vi "genHelpFileIn.vi"(0 "Output Cluster":T1) -> (5 "Help Description":string="\n")   [LabVIEW 2017]
uses:
  <vilib>/express/express shared/propPageData.ctl
panel:
  in  "Start Row Data":string="Start Row Data:"
  in  "Samples":string="Samples:"
  in  "File Path":string="File Path:"
  in  "Attempt to Read Generic Text Files enum":string[](array[string])=["False", "True"]
  in  "Attempt to Read Generic Text Files":string="Read Generic Text Files:"
  in  "Lock File enum":string[](array[string])=[" False", " True"]
  in  "Lock File":string="Lock File:"
  in  "First Column enum":string[](array[string])=[" False", " True"]
  in  "First Column is Time Channel":string="First Column is Time  Channel: "
  in  "First Row enum":string[](array[string])=[" False", " True"]
  in  "First Row is Channel Names:":string="First Row is Channel: Names:"
  in  "Segment Size enum":string[](array[string])=["Retrieve segments of original size", "Retrieve segments of specified size"]
  in  "Segment Size":string="Segment Size: "
  in  "File_dialog enum":string[](array[string])=[" False", " True"]
  in  "File_dialog":string="Ask User To Choose File:"
  in  "Decimal enum":string[](array[string])=[". (dot)", ". (comma)"]
  in  "Decimal":string="Decimal Point: "
  in  "Timestamp":string="Timestamp: "
  in  "Timestamp enum":string[](array[string])=["Absolute", "Relative"]
  in  "Delimiter enum":string[](array[string])=["Tabulator", "Comma"]
  in  "Delimiter":string="Delimiter: "
  in  "Format enum":string[](array[string])=["Text (LVM)", "Binary with XML Header (TDM)", "Binary (TDMS)"]
  in  "Format":string="File Format: "
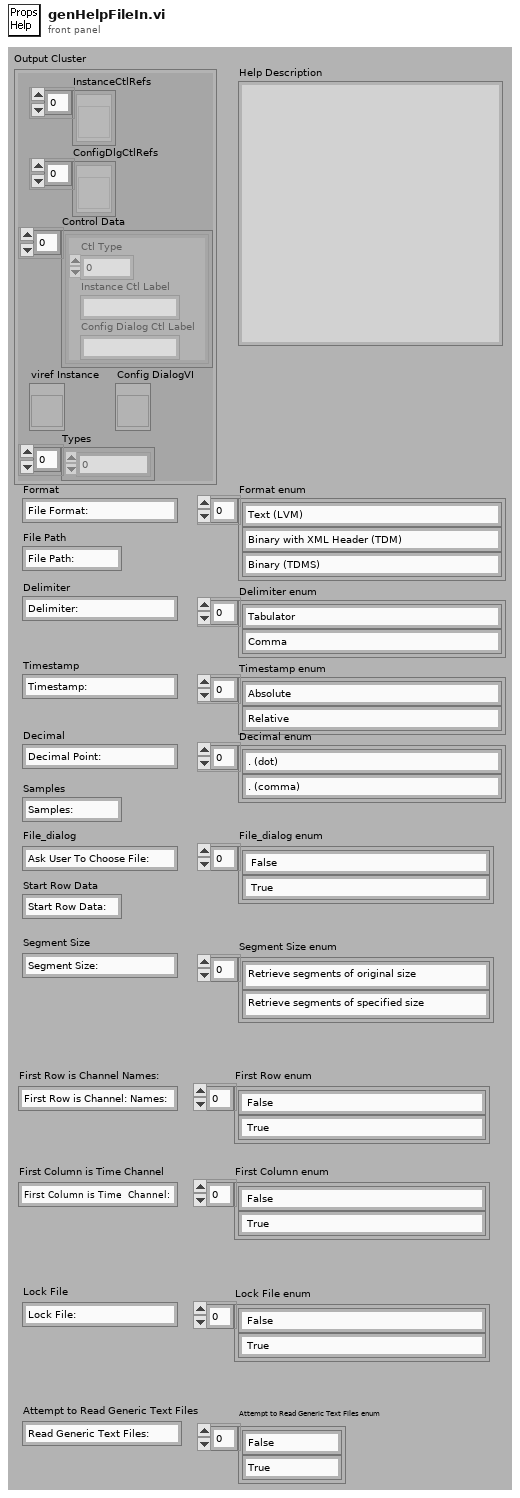
[diagram p1: front panel]
types:
  T1 = typedef "propPageData.ctl" = cluster{"InstanceCtlRefs":refnum<vi>[], "ConfigDlgCtlRefs":refnum<vi>[], "Control Data":cluster{"Ctl Type":u16, "Instance Ctl Label":string, "Config Dialog Ctl Label":string}[], "viref Instance":refnum<vi>, "Types":i32[], "Config DialogVI":refnum<vi>}
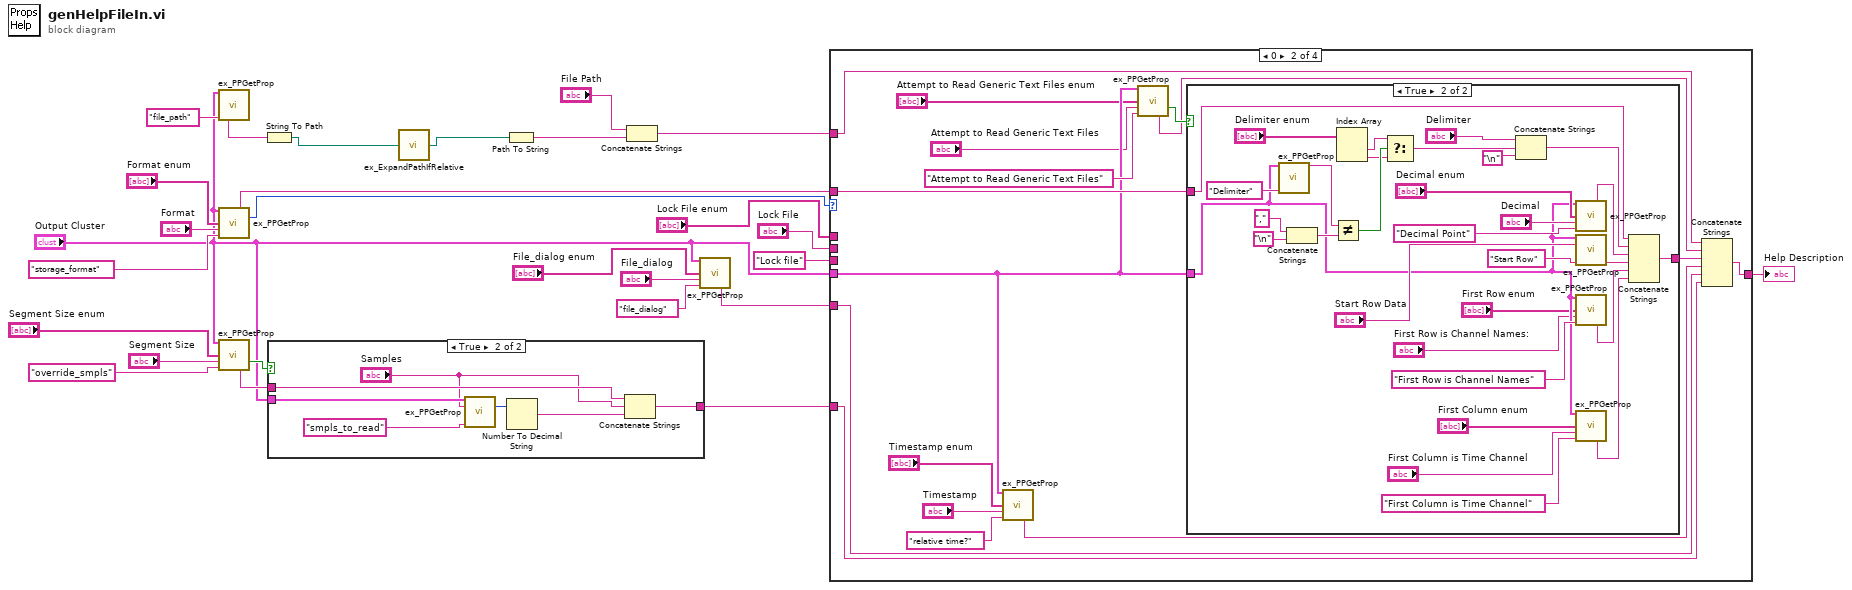
[diagram p0: block diagram]
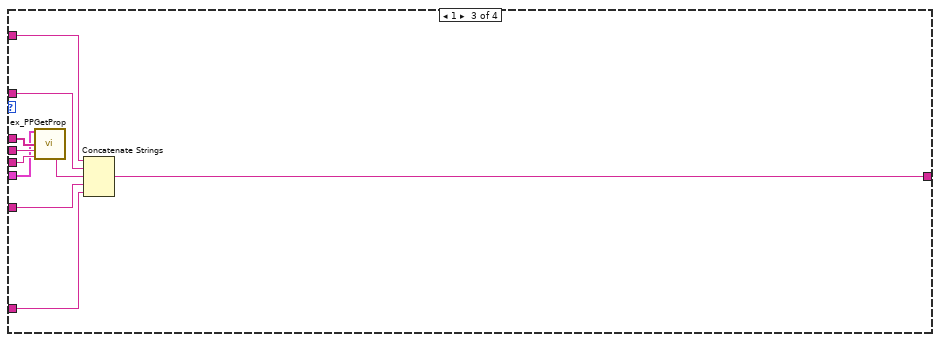
[diagram p5: hidden frame]
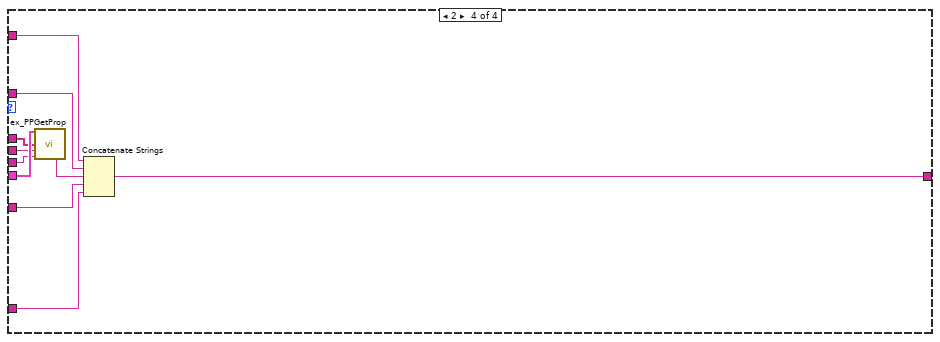
[diagram p6: hidden frame]
diagram:
  n1 = call <vilib>:"ex_PPGetProp.vi"("Output Cluster"="Output Cluster", "Control:"="file_path") -> ("String (Path)"=w6:string)  [unwired: 5 in, 8 out]
  n2 = call <vilib>:"ex_PPGetProp.vi"("Output Cluster"="Output Cluster", "Enum & T/F Strings"="Format enum", "Prefix"="Format", "Control:"="storage_format") -> ("Enum Result"=w24:string, "int32"=w23:i32)  [unwired: 3 in, 7 out]
  n3 = call <vilib>:"ex_PPGetProp.vi"("Output Cluster"="Output Cluster", "Enum & T/F Strings"="Segment Size enum", "Prefix"="Segment Size", "Control:"="override_smpls") -> ("bool"=w14:bool, "T/F Result"=w13:string)  [unwired: 3 in, 7 out]
  n4 = String To Path(string=w6) -> (path=w2:path)
  n5 = case shown="True" w14 {
    tunnel: [w28 w30] -> w12
    tunnel: w13 -> [w28 w32]
    tunnel: "Output Cluster" -> [_ w34]
    frame False {
    }
    frame True {
      n6 = call <vilib>:"ex_PPGetProp.vi"("Output Cluster"=w34, "Previous String"="Samples", "Control:"="smpls_to_read") -> ("int32"=w33:i32)  [unwired: 4 in, 8 out]
      n7 = Number To Decimal String(number=w33) -> (decimal integer string=w31:string)  [unwired: 1 in]
      n8 = Concatenate Strings(w32, "Samples", w31) -> (w30:string)
    }
  }
  n9 = call <vilib>:"ex_ExpandPathIfRelative.vi"("Path"=w2) -> ("Expanded path"=w1:path)  [unwired: 3 in, 1 out]
  n10 = Path To String(path=w1) -> (string=w5:string)
  n11 = Concatenate Strings("File Path", w5) -> (w3:string)
  n12 = call <vilib>:"ex_PPGetProp.vi"("Output Cluster"="Output Cluster", "Enum & T/F Strings"="File_dialog enum", "Prefix"="File_dialog", "Control:"="file_dialog") -> ("T/F Result"=w18:string)  [unwired: 3 in, 8 out]
  n13 = case shown="0" w23 {
    tunnel: "Output Cluster" -> [_ w44 w91 w104]
    tunnel: w24 -> [w36 w47 w90 w103]
    tunnel: [w36 w45 w86 w99] -> w22
    tunnel: w18 -> [_ w42 w88 w101]
    tunnel: w12 -> [_ w41 w87 w100]
    tunnel: "Lock File enum" -> [_ _ w94 w98]
    tunnel: "Lock File" -> [_ _ w93 w97]
    tunnel: "Lock file" -> [_ _ w92 w96]
    tunnel: w3 -> [_ w38 w85 w95]
    frame Default {
    }
    frame 0 {
      n14 = call <vilib>:"ex_PPGetProp.vi"("Output Cluster"=w44, "Enum & T/F Strings"="Timestamp enum", "Prefix"="Timestamp", "Control:"="relative time?") -> ("T/F Result"=w43:string)  [unwired: 3 in, 8 out]
      n15 = call <vilib>:"ex_PPGetProp.vi"("Output Cluster"=w44, "Enum & T/F Strings"="Attempt to Read Generic Text Files enum", "Prefix"="Attempt to Read Generic Text Files", "Control:"="Attempt to Read Generic Text Files") -> ("bool"=w51:bool, "T/F Result"=w37:string)  [unwired: 3 in, 7 out]
      n16 = case shown="True" w51 {
        tunnel: w44 -> [_ w60]
        tunnel: w47 -> [w53 w81]
        tunnel: [w53 w80] -> w46
        frame False {
        }
        frame True {
          n17 = call <vilib>:"ex_PPGetProp.vi"("Output Cluster"=w60, "Control:"="Delimiter") -> ("String"=w70:string)  [unwired: 5 in, 8 out]
          n18 = Concatenate Strings("," ("y"), "\n") -> (w69:string)
          n19 = Not Equal?(x=w70, y=w69) -> (x != y?=w77:bool)
          n20 = Index Array(array="Delimiter enum") -> (element #1=w75:string, element #2=w74:string)  [unwired: 2 in]
          n21 = Select(t=w75, s=w77, f=w74) -> (s? t:f=w73:string)
          n22 = Concatenate Strings("Delimiter", w73, "\n") -> (w71:string)
          n23 = call <vilib>:"ex_PPGetProp.vi"("Output Cluster"=w60, "Enum & T/F Strings"="Decimal enum", "Prefix"="Decimal", "Control:"="Decimal Point") -> ("Enum Result"=w79:string)  [unwired: 3 in, 8 out]
          n24 = call <vilib>:"ex_PPGetProp.vi"("Output Cluster"=w60, "Previous String"="Start Row Data", "Control:"="Start Row") -> ("dbl String"=w64:string)  [unwired: 4 in, 8 out]
          n25 = call <vilib>:"ex_PPGetProp.vi"("Output Cluster"=w60, "Enum & T/F Strings"="First Row enum", "Prefix"="First Row is Channel Names:", "Control:"="First Row is Channel Names") -> ("T/F Result"=w61:string)  [unwired: 3 in, 8 out]
          n26 = call <vilib>:"ex_PPGetProp.vi"("Output Cluster"=w60, "Enum & T/F Strings"="First Column enum", "Prefix"="First Column is Time Channel", "Control:"="First Column is Time Channel") -> ("T/F Result"=w54:string)  [unwired: 3 in, 8 out]
          n27 = Concatenate Strings(w81, w71, w79, w64, w61, w54) -> (w80:string)
        }
      }
      n28 = Concatenate Strings(w38, w37, w46, w43, w42, w41) -> (w45:string)
    }
    frame 1 {
      n29 = call <vilib>:"ex_PPGetProp.vi"("Output Cluster"=w91, "Enum & T/F Strings"=w94, "Prefix"=w93, "Control:"=w92) -> ("T/F Result"=w89:string)  [unwired: 3 in, 8 out]
      n30 = Concatenate Strings(w85, w90, w89, w88, w87) -> (w86:string)
    }
    frame 2 {
      n31 = call <vilib>:"ex_PPGetProp.vi"("Output Cluster"=w104, "Enum & T/F Strings"=w98, "Prefix"=w97, "Control:"=w96) -> ("T/F Result"=w102:string)  [unwired: 3 in, 8 out]
      n32 = Concatenate Strings(w95, w103, w102, w101, w100) -> (w99:string)
    }
  }
  "Help Description" <- w22
